vi "Test MQTT-3.2.2-2.vi"(8 "error in (no error)":errorcluster, 11 "Connection Config":refnum<class "Connection.lvclass">) -> (0 "error out":errorcluster, 3 "Connection Config dup":refnum<class "Connection.lvclass">)   [LabVIEW 2013]
uses:
  <vilib>/LabVIEW Open Source Project/MQTT Connection/MQTT_Connection/Connection/Connection.lvclass
  <vilib>/LabVIEW Open Source Project/MQTT Control Packets/Control Packets/CONNECT/ConnectFlags -- cluster.ctl
  <vilib>/LabVIEW Open Source Project/MQTT Control Packets/Control Packets/CONNECT/CONNECT.lvclass
  <vilib>/LabVIEW Open Source Project/MQTT Control Packets/Control Packets/ControlPacket/ControlPacket.lvclass
  <vilib>/addons/_JKI Toolkits/Caraya/classes/Test/Test.lvclass
  <vilib>/LabVIEW Open Source Project/MQTT Control Packets/Control Packets/DISCONNECT/DISCONNECT.lvclass
  <vilib>/addons/_JKI Toolkits/Caraya/classes/Assert/Assert.lvclass
panel:
  out "Bytes 2":u8[](array[numeric]) format="%08b"
  out "Bytes":u8[](array[numeric]) format="%08b"
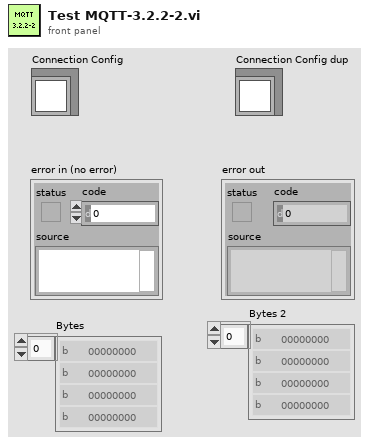
[diagram p1: front panel]
types:
  T1 = typedef "MQTT_Control_Packets.lvlib/CONNECT.lvclass/ConnectFlags -- cluster.ctl" = cluster{"Reserved":bool, "Clean Session":bool, "Will Flag":bool, "Will QoS 1":bool, "Will QoS 2":bool, "Will Retain":bool, "Password Flag":bool, "User Name Flag":bool}
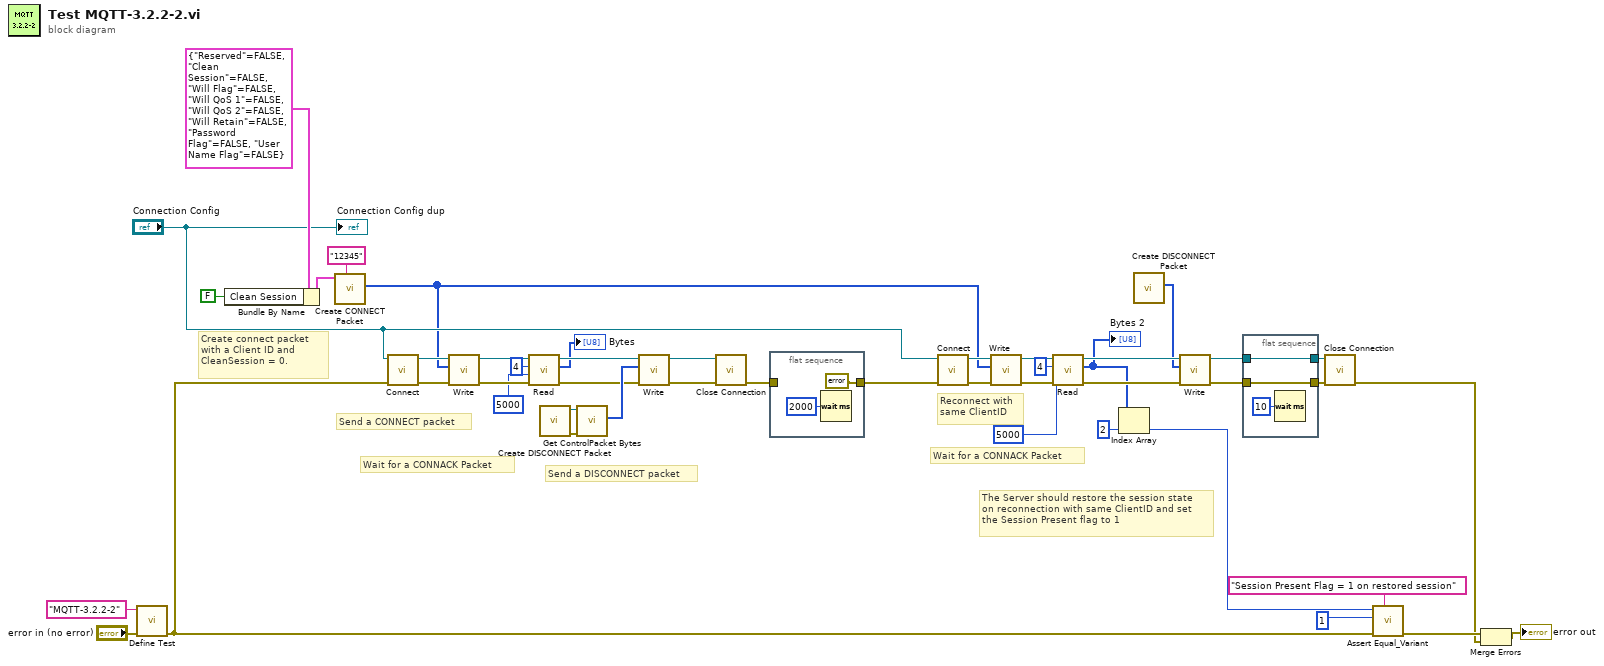
[diagram p0: block diagram]
diagram:
  # "Wait for a CONNACK Packet"
  # "The Server should restore the session state\non reconnection with same ClientID and set\nthe Session Present flag to 1"
  # "Reconnect with\nsame ClientID"
  # "Send a DISCONNECT packet"
  # "Wait for a CONNACK Packet"
  # "Create connect packet with a Client ID and CleanSession = 0."
  # "Send a CONNECT packet"
  n1 = call <vilib>:"Define Test.vi"("error in (no error)"="error in (no error)", "Label (VI Title)"="MQTT-3.2.2-2") -> ("error out"=w12:errorcluster)  [unwired: 9 in]
  n2 = Bundle By Name(cluster=T1 {"Reserved"=FALSE, "Clean Session"=FALSE, "Will Flag"=FALSE, "Will QoS 1"=FALSE, "Will QoS 2"=FALSE, "Will Retain"=FALSE, "Password Flag"=FALSE, "User Name Flag"=FALSE} ("Connect Flags"), "Clean Session"=FALSE) -> (w33:T1)
  n3 = call <vilib>:"Create CONNECT Packet.vi"("Client ID (empty: generate new)"="12345", "Connect Flags"=w33) -> ("Bytes Stream"=w1:u8[])  [unwired: 7 in, 2 out]
  n4 = call <vilib>:"Connect.vi"("error in (no error)"=w12, "Connection in"="Connection Config") -> ("error out"=w31:errorcluster, "Connection out"=w30:refnum<class "Connection.lvclass">)  [unwired: 8 in]
  n5 = call <vilib>:"Write.vi"("error in (no error)"=w31, "Bytes"=w1, "Connection in"=w30) -> ("error out"=w37:errorcluster, "Connection"=w38:refnum<class "Connection.lvclass">)  [unwired: 7 in]
  n6 = call <vilib>:"Read.vi"("error in (no error)"=w37, "timeout (2000 ms)"=5000 ("timeout (1000 ms)"), "bytes to read (100)"=4 ("bytes to read"), "TCPConnection in"=w38) -> ("error out"=w23:errorcluster, "Bytes"=→"Bytes":u8[], "TCPConnection out"=w24:refnum<class "Connection.lvclass">)  [unwired: 3 in, 2 out]
  n7 = call <vilib>:"Create DISCONNECT Packet.vi"() -> ("error out"=w43:errorcluster, "DISCONNECT"=w42:refnum<class "DISCONNECT.lvclass">)  [unwired: 9 in, 1 out]
  n8 = call <vilib>:"Get ControlPacket Bytes.vi"("error in (no error)"=w43, "ControlPacket"=w42) -> ("Bytes Stream"=w41:u8[])  [unwired: 6 in, 3 out]
  n9 = call <vilib>:"Write.vi"("error in (no error)"=w23, "Bytes"=w41, "Connection in"=w24) -> ("error out"=w9:errorcluster, "Connection"=w10:refnum<class "Connection.lvclass">)  [unwired: 7 in]
  n10 = call <vilib>:"Close Connection.vi"("error in (no error)"=w9, "Connection in"=w10) -> ("error out"=w8:errorcluster)  [unwired: 8 in, 1 out]
  n11 = flat-sequence {
    tunnel: [errorcluster {"status"=FALSE, "code"=0, "source"=""} ("error out")] -> w7
    tunnel: w8 -> [_]
    frame #0 {
      n12 = Wait (ms)(milliseconds to wait=u32 2000) -> ()  [unwired: 1 out]
    }
  }
  n13 = call <vilib>:"Connect.vi"("error in (no error)"=w7, "Connection in"="Connection Config") -> ("error out"=w29:errorcluster, "Connection out"=w28:refnum<class "Connection.lvclass">)  [unwired: 8 in]
  n14 = call <vilib>:"Write.vi"("error in (no error)"=w29, "Bytes"=w1, "Connection in"=w28) -> ("error out"=w25:errorcluster, "Connection"=w26:refnum<class "Connection.lvclass">)  [unwired: 7 in]
  n15 = call <vilib>:"Read.vi"("error in (no error)"=w25, "timeout (2000 ms)"=5000 ("timeout (1000 ms)"), "bytes to read (100)"=4 ("bytes to read"), "TCPConnection in"=w26) -> ("error out"=w19:errorcluster, "Bytes"=w5:u8[], "TCPConnection out"=w18:refnum<class "Connection.lvclass">)  [unwired: 3 in, 2 out]
  "Bytes 2" <- w5
  n16 = Index Array(array=w5, index=2) -> (element=w22:u8)
  n17 = call <vilib>:"Create DISCONNECT Packet.vi"() -> ("Bytes Stream"=w2:u8[])  [unwired: 9 in, 2 out]
  n18 = call <vilib>:"Write.vi"("error in (no error)"=w19, "Bytes"=w2, "Connection in"=w18) -> ("error out"=w15:errorcluster, "Connection"=w14:refnum<class "Connection.lvclass">)  [unwired: 7 in]
  n19 = flat-sequence {
    tunnel: w14 -> [w51]
    tunnel: [w51] -> w16
    tunnel: [w49] -> w17
    tunnel: w15 -> [w49]
    frame #0 {
      n20 = Wait (ms)(milliseconds to wait=u32 10) -> ()  [unwired: 1 out]
    }
  }
  n21 = call <vilib>:"Close Connection.vi"("error in (no error)"=w17, "Connection in"=w16) -> ("error out"=w13:errorcluster)  [unwired: 8 in, 1 out]
  n22 = call <vilib>:"Assert Equal_Variant.vi"("Label"="Session Present Flag = 1 on restored session", "error in (no error)"=w12, "Y"=u8 1 ("element"), "X"=w22) -> ("error out"=w35:errorcluster)  [unwired: 7 in]
  n23 = Merge Errors(w35, w13) -> (→"error out":errorcluster)
  "Connection Config dup" <- "Connection Config"
